vi "Import Configuration RTM.vi"(8 "error in (no error)":errorcluster, 11 "Node Ptr":u64 format="%.0x") -> (0 "error out":errorcluster)   [LabVIEW 2020, in "Ballard MIL-STD-1553 System Explorer.lvlib" / "Implementation.lvlib"]
uses:
  Implementation.lvlib
  Scripting/Custom Device/Import Custom Device (In Place).vi
  Scripting/Ballard MIL-STD-1553 Scripting.lvlib
panel:
  in  "Tag":string
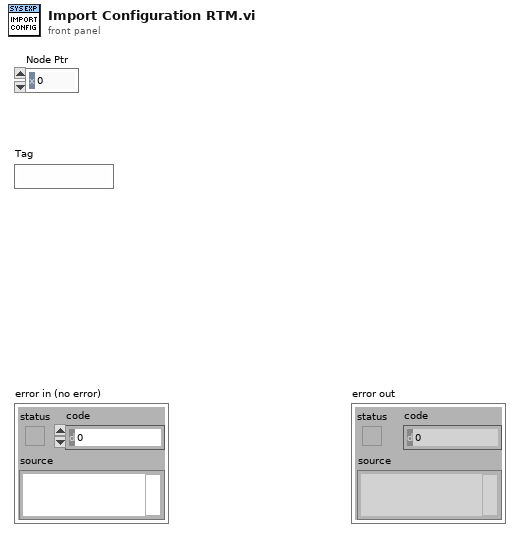
[diagram p1: front panel]
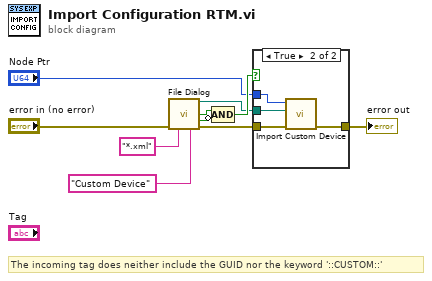
[diagram p0: block diagram]
diagram:
  # "The incoming tag does neither include the GUID nor the keyword '::CUSTOM::'"
  n1 = call "File Dialog"("error in"="error in (no error)", "pattern (all files)"="*.xml" ("pattern label"), "pattern label"="Custom Device") -> ("selected path"=w2:path, "exists"=w7:bool, "cancelled"=w6:bool, "error out"=w4:errorcluster)  [unwired: 9 in]
  n2 = Compound Arithmetic op=AND(w7, invert w6) -> (w5:bool)
  n3 = case shown="True" w5 {
    tunnel: w4 -> [w11 w13]
    tunnel: "Node Ptr" -> [_ w15]
    tunnel: w2 -> [_ w14]
    tunnel: [w11 w12] -> w1
    frame False {
    }
    frame True {
      n4 = call-poly "Import Custom Device.vi"("error in"=w13, "path"=w14, "custom device ref"=w15) -> ("error out"=w12:errorcluster)  [unwired: 7 in, 1 out]
    }
  }
  "error out" <- w1
